vi "Time Keeper.vi"(8 "Reset?":bool) -> (3 "Time Elapsed (ms)":u32)   [LabVIEW 2017]
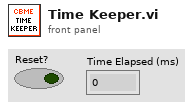
[diagram p1: front panel]
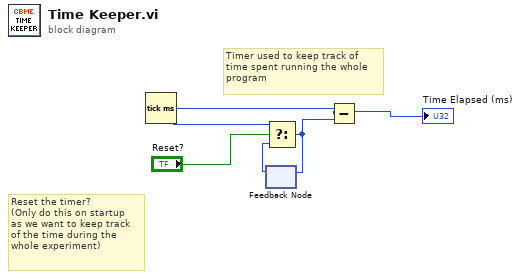
[diagram p0: block diagram]
diagram:
  # "Reset the timer?\n(Only do this on startup\nas we want to keep track \nof the time during the \nwhole experiment)"
  # "Timer used to keep track of\ntime spent running the whole\nprogram"
  n1 = Tick Count (ms)() -> (millisecond timer value=w5:u32)
  n2 = feedback #1() -> (w3:u32)  [unwired: 1 in]
  n3 = Select(t=w5, s="Reset?", f=w3) -> (s? t:f=w2:u32)
  n4 = feedback-in #1(w2) -> ()
  n5 = Subtract(x=w5, y=w2) -> (x-y=→"Time Elapsed (ms)":u32)
